vi "Exit.vi"(8 "error in (no error)":errorcluster, 11 "Old State":refnum<class "Command State Actor.lvclass">) -> (0 "error out":errorcluster, 3 "New State":refnum<class "Command State Actor.lvclass">)   [LabVIEW 2013, in "Command State Actor.lvlib" / "Command State Actor.lvclass"]
doc: "This is an abstract method. Override this method to define the behavior when you leave the state."
uses:
  Command State Actor.lvclass
  <vilib>/ni/Actors/State Actor/State Actor/State Actor.lvclass
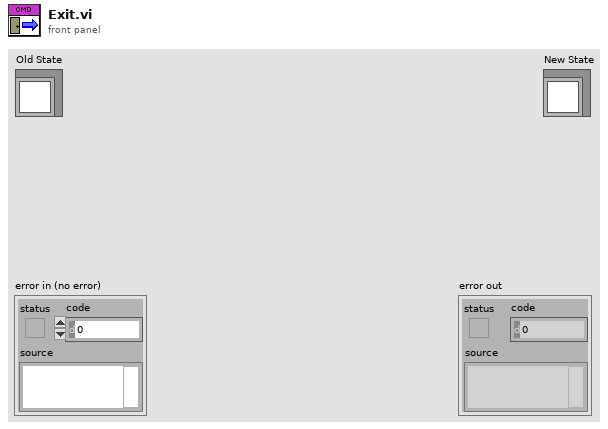
[diagram p1: front panel]
types:
  T1 = typedef "Command State Actor.lvlib/Command State Actor.lvclass/Command Status.ctl" = cluster{"CurrentCommandState":T2, "Command Name":string, "Current State Status":T3, "Command Start Time":timestamp, "Command End Time":timestamp, "Previous State Status":T3}
  T2 = typedef "Command State Actor.lvlib/Command State Actor.lvclass/Command States.ctl" = enum16{"NotStarted", "Starting", "Started", "Executing", "Completing", "Completed", "Stopping", "Stopped"}
  T3 = typedef "Command Actor.lvlib/Command States.lvclass/State Status.ctl" = cluster{"State Name":string, "State Entry Time":timestamp, "State Exit Time":timestamp}
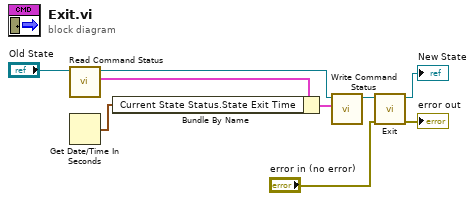
[diagram p0: block diagram]
diagram:
  n1 = call-dynamic "Read Command Status.vi"("Command in"="Old State") -> ("Command Status"=w3:T1, "Command out"=w5:refnum<class "Command State Actor.lvclass">)  [unwired: 8 in, 1 out]
  n2 = Get Date/Time In Seconds() -> (seconds since 1Jan1904=w1:timestamp)
  n3 = Bundle By Name(cluster=w3, "Current State Status.State Exit Time"=w1) -> (w2:T1)
  n4 = call-dynamic "Write Command Status.vi"("Command Status"=w2, "Command in"=w5) -> ("Command out"=w4:refnum<class "Command State Actor.lvclass">)  [unwired: 8 in, 1 out]
  n5 = call-parent "Exit.vi"("error in (no error)"="error in (no error)", "Old State"=w4) -> ("error out"=→"error out":errorcluster, "New State"=→"New State":refnum<class "Command State Actor.lvclass">)  [unwired: 8 in]
